vi "Splash Obtain Queue.vi"(8 "error in (no error)":errorcluster, 11 "name":string) -> (0 "error out":errorcluster, 3 "splash queue out":refnum<queue>)   [LabVIEW 2013, in "SET_Splash.lvlib"]
uses:
  SET_Splash.lvlib
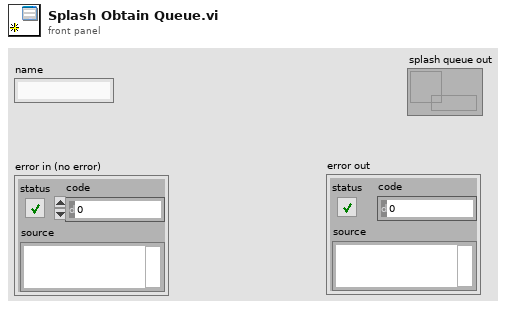
[diagram p1: front panel]
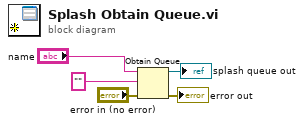
[diagram p0: block diagram]
diagram:
  n1 = Obtain Queue(name (unnamed)="name", element data type="", error in (no error)="error in (no error)") -> (queue out=→"splash queue out":refnum<queue>, error out=→"error out":errorcluster)  [unwired: 2 in, 1 out]
